vi "Rename Object Labels.vi"(6 "Post":string, 8 "error in":errorcluster, 9 "Pre":string, 10 "Class Ref":refnum<vi>) -> (0 "error out":errorcluster)   [LabVIEW 2025, in "_Rename.lvlib" / "_Rename.lvclass"]
uses:
  _Rename.lvclass
  _Rename.lvclass/_Rename.ctl
  <vilib>/Utility/traverseref.llb/TRef TravTarget.ctl
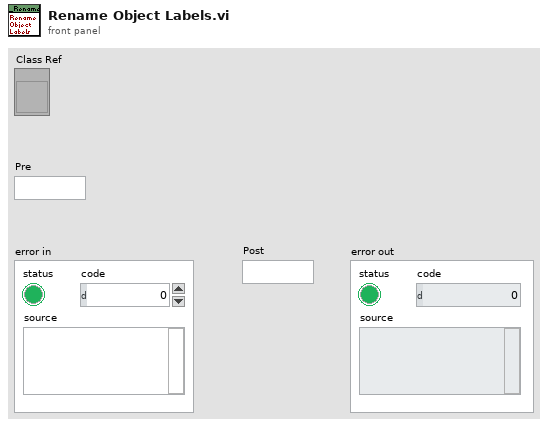
[diagram p1: front panel]
types:
  T1 = typedef "TRef TravTarget.ctl" = enum16{"FP", "BD", "Other"}
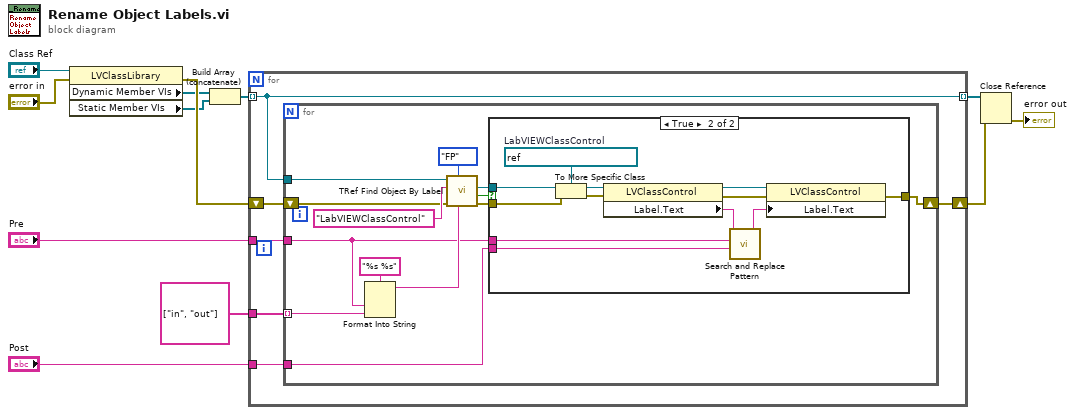
[diagram p0: block diagram]
diagram:
  n1 = property class="LVClassLibrary"(reference="Class Ref", error in="error in") -> (error out=w12:errorcluster, "Dynamic Member VIs"=w9:refnum<vi>[], "Static Member VIs"=w10:refnum<vi>[])  [unwired: 1 out]
  n2 = Build Array (concatenate)(w9, w10) -> (w11:refnum<vi>[])
  n3 = for {
    tunnel: w11 -> [w17] mode=indexing
    shift-right: [w16] -> w7
    shift-left: w12 -> [w18]
    tunnel: [w17] -> w8 mode=indexing
    tunnel: "Pre" -> [w15]
    tunnel: "Post" -> [w14]
    tunnel: string[] ["in", "out"] -> [w13]
    n4 = for {
      tunnel: w17 -> [w24]
      tunnel: w13 -> [w22] mode=indexing
      shift-right: [w21] -> w16
      shift-left: w18 -> [w23]
      tunnel: w15 -> [w20]
      tunnel: w14 -> [w19]
      n5 = Format Into String(format string="%s %s", w20, w22) -> (resulting string=w29:string)  [unwired: 2 in, 1 out]
      n6 = call <vilib>:"TRef Find Object By Label.vi"("Label"=w29, "Traverse Target"=TRef_TravTarget."FP", "error in (no error)"=w23, "Class Name"="LabVIEWClassControl", "VI Ref"=w24) -> ("error out"=w28:errorcluster, "Found?"=w27:bool, "Found Obj Ref"=w31:refnum<vi>)  [unwired: 3 in, 1 out]
      n7 = case shown="True" w27 {
        tunnel: [_ w43] -> w21
        tunnel: w31 -> [_ w41]
        tunnel: w28 -> [_ w42]
        tunnel: w20 -> [_ w33]
        tunnel: w19 -> [_ w32]
        frame False {
          # "The \"in\" or \"out\" doesn't exist so..\ndo nothing"
        }
        frame True {
          w40 = refnum<vi> refnum  # LabVIEWClassControl
          n8 = To More Specific Class(target class=w40, reference=w41, error in=w42) -> (specific class reference=w39:refnum<vi>, error out=w38:errorcluster)
          n9 = property class="LVClassControl"(reference=w39, error in=w38) -> (reference out=w36:refnum<vi>, error out=w37:errorcluster, "Label.Text"=w35:string)
          n10 = call <vilib>:"Search and Replace Pattern.vi"("string"=w35, "regular expression (\"\")"=w33, "replace string (\"\")"=w32) -> ("result string"=w34:string)  [unwired: 2 in, 1 out]
          n11 = property class="LVClassControl"(reference=w36, error in=w37, "Label.Text"=w34) -> (error out=w43:errorcluster)  [unwired: 1 out]
        }
      }
    }
  }
  n12 = Close Reference(reference=w8, error in (no error)=w7) -> (error out=→"error out":errorcluster)
